vi "Problem2.7.vi"() -> ()   [LabVIEW 2019]
panel:
  out "Changed Quantity":dbl
  out "Elapsed Time (s)":dbl
  out "Speed  Chart":dbl(graph)
  out "Rate of Change":dbl
  in  "Changed Quantity":dbl(slide) scale=0.0..100.0
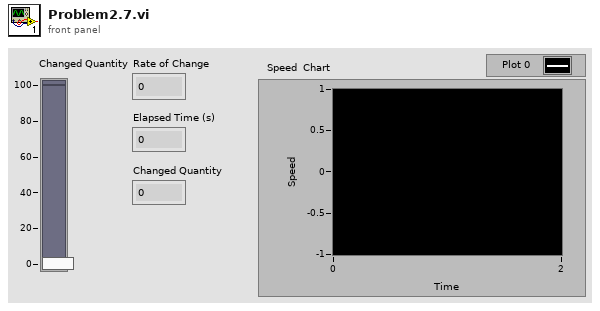
[diagram p1: front panel]
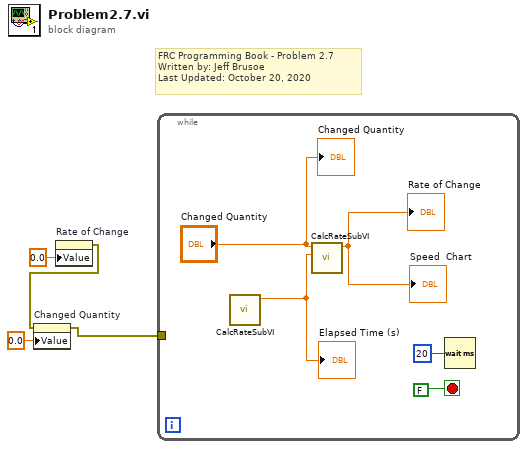
[diagram p0: block diagram]
diagram:
  # "FRC Programming Book - Problem 2.7\nWritten by: Jeff Brusoe\nLast Updated: October 20, 2020"
  n1 = property on="Rate of Change" class="DigNum (strict)"("Value"=0.0 ("Rate of Change")) -> (error out=w2:errorcluster)  [unwired: 2 in, 1 out]
  n2 = property on="Changed Quantity" class="Slide (strict)"(error in=w2, "Value"=0.0 ("Changed Quantity")) -> (error out=w1:errorcluster)  [unwired: 1 in, 1 out]
  n3 = while {
    tunnel: w1 -> [_]
    stop <- FALSE stop-if-true
    n4 = call "CalcRateSubVI.vi"() -> ("Rate of Change"=w5:dbl)  [unwired: 11 in]
    "Elapsed Time (s)" <- w5
    n5 = call "CalcRateSubVI.vi"("Elapsed Time (s)"=w5, "Changed Quantity"="Changed Quantity") -> ("Rate of Change"=→"Speed  Chart" →"Rate of Change":dbl)  [unwired: 9 in]
    n6 = Wait (ms)(milliseconds to wait=u32 20) -> ()  [unwired: 1 out]
    "Changed Quantity" <- "Changed Quantity"
  }
